vi "TCPPacket Read Body.vi"(8 "error in (no error)":errorcluster, 10 "Data":u8[](array[numeric]), 11 "TCPPacket in":refnum<class "TCPPacket.lvclass">) -> (0 "error out":errorcluster, 3 "TCPPacket out":refnum<class "TCPPacket.lvclass">)   [LabVIEW 2019, in "TCPPacket.lvclass"]
uses:
  TCPPacket.lvclass
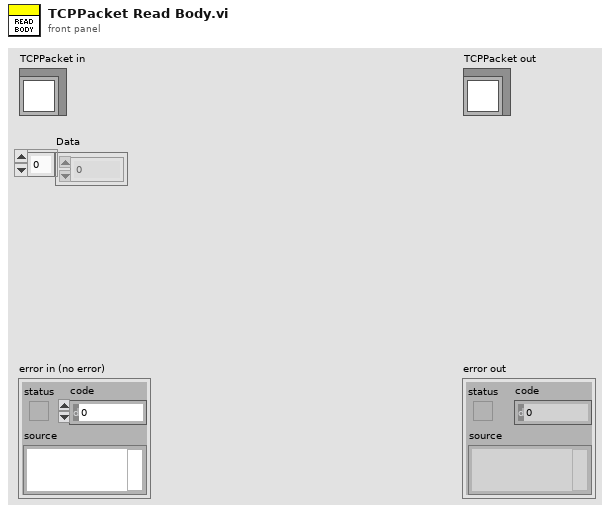
[diagram p1: front panel]
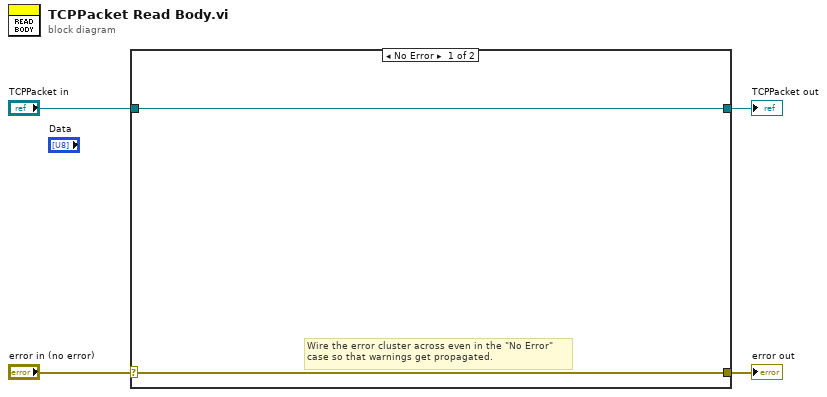
[diagram p0: block diagram]
diagram:
  n1 = case shown="No Error" "error in (no error)" {
    selector: "error in (no error)" -> [w5 w8]
    tunnel: [w5 w8] -> w3
    tunnel: [w6 w7] -> w1
    tunnel: "TCPPacket in" -> [w6 w7]
    frame No Error {
      # "Wire the error cluster across even in the \"No Error\"\ncase so that warnings get propagated."
    }
    frame Error {
    }
  }
  "error out" <- w3
  "TCPPacket out" <- w1
